vi "8 Ch Digital Input.vi"(2 "8 Ch Digital In":T1={"DI0"="Chassis1/Mod4/DI0", "DI1"="Chassis1/Mod4/DI0", "DI2"="Chassis1/Mod4/DI0", "DI3"="Chassis1/Mod4/DI0", "DI4"="Chassis1/Mod4/DI0", "DI5"="Chassis1/Mod4/DI0", "DI6"="Chassis1/Mod4/DI0", "DI7"="Chassis1/Mod4/DI0"}) -> (7 "Packet":u64)   [LabVIEW 2009]
uses:
  <vilib>/eio/EIONode/EIONode.xnode
  <vilib>/rvi/eio/nirviEIOImplementation/nirviEIOImplementation.xnode
  <vilib>/rvi/eio/common/nirviEmuTemplateMethod_noerrors.vi
  <vilib>/rvi/eio/common/nirviEmuClasses.ctl
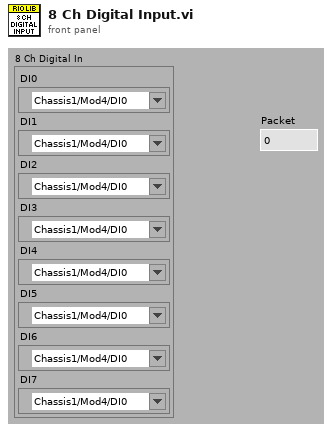
[diagram p1: front panel]
types:
  T1 = cluster{"DI0":refnum<k21>, "DI1":refnum<k21>, "DI2":refnum<k21>, "DI3":refnum<k21>, "DI4":refnum<k21>, "DI5":refnum<k21>, "DI6":refnum<k21>, "DI7":refnum<k21>}
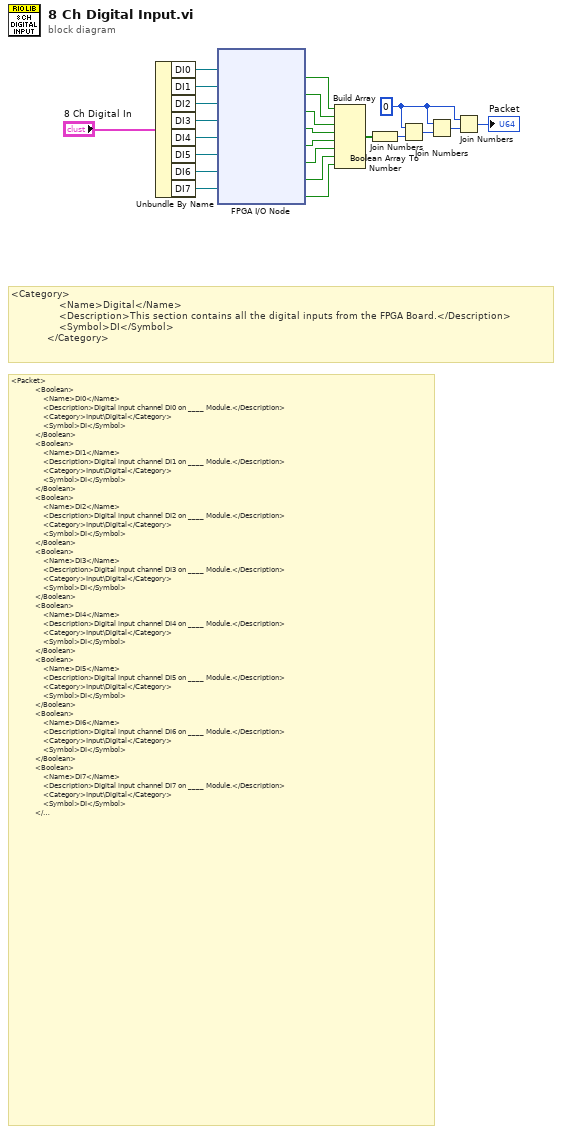
[diagram p0: block diagram]
diagram:
  w9 = u8 0 ("hi")
  # "<Category>\n                <Name>Digital</Name>\n                <Description>This section contains all the digital inputs from the FPGA Board.</Description>\n                <Symbol>DI</Symbol>\n            </Category>"
  # "<Packet>\n            <Boolean>\n                <Name>DI0</Name>\n                <Description>Digital input channel DI0 on ____ Module.</Description>\n                <Category>Input\\Digital</Category>\n                <Symbol>DI</Symbol>\n            </Boolean>\n            <Boolean>\n                <Name>DI1</Name>\n                <Description>Digital input channel DI1 on ____ Module.</Description>\n                <Category>Input\\Digital</Category>\n                <Symbol>DI</Symbol>\n            </Boolean>\n            <Boolean>\n                <Name>DI2</Name>\n                <Description>Digital input channel DI2 on ____ Module.</Description>\n                <Category>Input\\Digital</Category>\n                <Symbol>DI</Symbol>\n            </Boolean>\n            <Boolean>\n                <Name>DI3</Name>\n                <Description>Digital input channel DI3 on ____ Module.</Description>\n                <Category>Input\\Digital</Category>\n                <Symbol>DI</Symbol>\n            </Boolean>\n            <Boolean>\n                <Name>DI4</Name>\n                <Description>Digital input channel DI4 on ____ Module.</Description>\n                <Category>Input\\Digital</Category>\n                <Symbol>DI</Symbol>\n            </Boolean>\n            <Boolean>\n                <Name>DI5</Name>\n                <Description>Digital input channel DI5 on ____ Module.</Description>\n                <Category>Input\\Digital</Category>\n                <Symbol>DI</Symbol>\n            </Boolean>\n            <Boolean>\n                <Name>DI6</Name>\n                <Description>Digital input channel DI6 on ____ Module.</Description>\n                <Category>Input\\Digital</Category>\n                <Symbol>DI</Symbol>\n            </Boolean>\n            <Boolean>\n                <Name>DI7</Name>\n                <Description>Digital input channel DI7 on ____ Module.</Description>\n                <Category>Input\\Digital</Category>\n                <Symbol>DI</Symbol>\n            </Boolean>\n        </Packet>"
  n1 = Unbundle By Name("8 Ch Digital In") -> ("DI0"=w20:refnum<k21>, "DI1"=w23:refnum<k21>, "DI2"=w22:refnum<k21>, "DI3"=w21:refnum<k21>, "DI4"=w5:refnum<k21>, "DI5"=w6:refnum<k21>, "DI6"=w7:refnum<k21>, "DI7"=w8:refnum<k21>)
  n2 = xnode "FPGA I/O Node"("FPGA I/O In"=w20, "FPGA I/O In"=w23, "FPGA I/O In"=w22, "FPGA I/O In"=w21, "FPGA I/O In"=w5, "FPGA I/O In"=w6, "FPGA I/O In"=w7, "FPGA I/O In"=w8) -> ("I/O Item"=w15:bool, "I/O Item"=w17:bool, "I/O Item"=w18:bool, "I/O Item"=w16:bool, "I/O Item"=w1:bool, "I/O Item"=w2:bool, "I/O Item"=w3:bool, "I/O Item"=w4:bool)  [unwired: 8 out]
  n3 = Build Array(w15, w17, w18, w16, w1, w2, w3, w4) -> (w14:bool[])
  n4 = Boolean Array To Number(Boolean array=w14) -> (number=w13:u8)
  n5 = Join Numbers(hi=w9, lo=w13) -> ((hi.lo)=w12:u16)
  n6 = Join Numbers(hi=w9, lo=w12) -> ((hi.lo)=w11:u32)
  n7 = Join Numbers(hi=w9, lo=w11) -> ((hi.lo)=→"Packet":u64)
